vi "Write Project Reference.vi"(8 "error in (no error)":errorcluster, 10 "Project Reference":refnum<vi>, 11 "MVA Comms VI in":refnum<class "MVA Comms VI Instance.lvclass">) -> (0 "error out":errorcluster, 3 "MVA Comms VI out":refnum<class "MVA Comms VI Instance.lvclass">)   [LabVIEW 2019, in "MVA Message Mapper.lvlib" / "MVA Comms VI Instance.lvclass"]
uses:
  <vilib>/gpm_packages/@cs/Bus-message-mapper/Source/support/MVA Comms/MVA Comms VI Instance.lvclass
  <vilib>/gpm_packages/@cs/Bus-message-mapper/Source/support/MVA Comms/MVA Comms VI Instance.lvclass/MVA Comms VI Instance.ctl
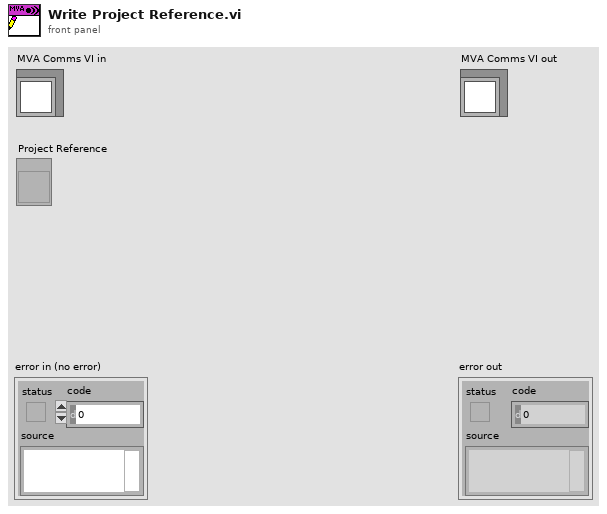
[diagram p1: front panel]
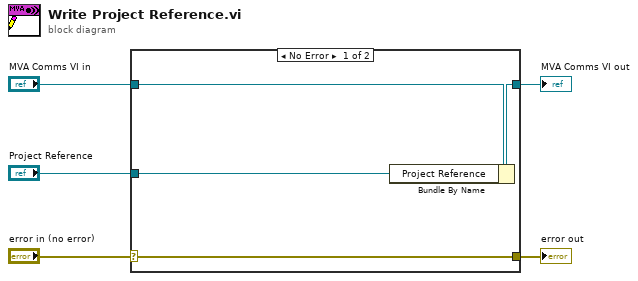
[diagram p0: block diagram]
diagram:
  n1 = case shown="No Error" "error in (no error)" {
    selector: "error in (no error)" -> [w9 w10]
    tunnel: [w9 w10] -> w4
    tunnel: [w7 w11] -> w2
    tunnel: "MVA Comms VI in" -> [w8 w11]
    tunnel: "Project Reference" -> [w6 _]
    frame No Error {
      n2 = Bundle By Name(cluster=w8, "Project Reference"=w6) -> (w7:refnum<class "MVA Comms VI Instance.lvclass">)
    }
    frame Error {
    }
  }
  "error out" <- w4
  "MVA Comms VI out" <- w2
